vi "write_params.vi"(8 "error in (no error)":errorcluster, 10 "params":T1={"priors"=[], "var_smoothing"=1e-09}, 11 "GaussianNB in":refnum<class "GaussianNB.lvclass">) -> (0 "error out":errorcluster, 3 "GaussianNB out":refnum<class "GaussianNB.lvclass">)   [LabVIEW 2020, in "GaussianNB.lvclass"]
uses:
  GaussianNB.lvclass
  Controls/gaussian_nb_params.ctl
  GaussianNB.lvclass/GaussianNB.ctl
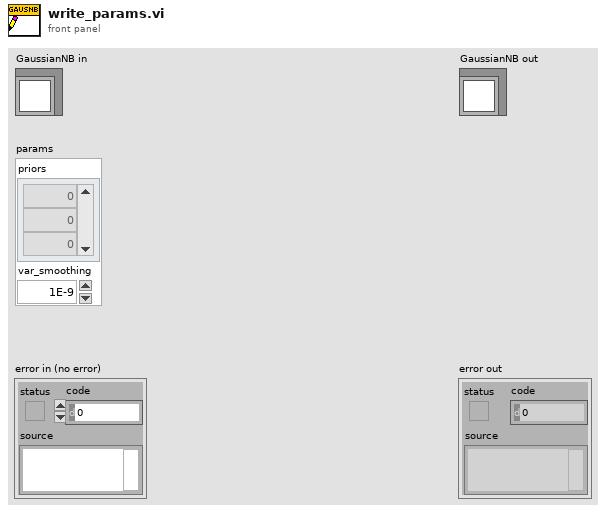
[diagram p1: front panel]
types:
  T1 = typedef "gaussian_nb_params.ctl" = cluster{"priors":dbl[], "var_smoothing":dbl}
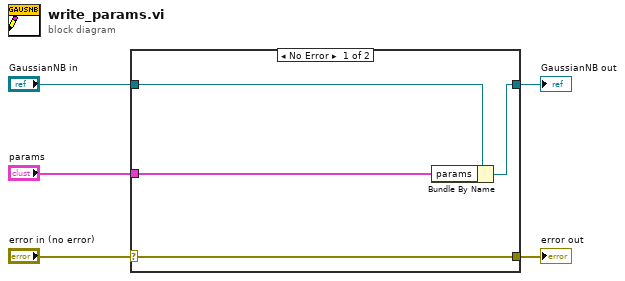
[diagram p0: block diagram]
diagram:
  n1 = case shown="No Error" "error in (no error)" {
    selector: "error in (no error)" -> [w9 w10]
    tunnel: [w9 w10] -> w4
    tunnel: [w7 w11] -> w2
    tunnel: "GaussianNB in" -> [w8 w11]
    tunnel: "params" -> [w6 _]
    frame No Error {
      n2 = Bundle By Name(cluster=w8, "params"=w6) -> (w7:refnum<class "GaussianNB.lvclass">)
    }
    frame Error {
    }
  }
  "error out" <- w4
  "GaussianNB out" <- w2
